vi "Fun gen and scope March 22 2017.vi"() -> ()   [LabVIEW 2014]
uses:
  <instrlib>/Tektronix TDS 200 1000 2000 Series/Public/Data/Read (Single Waveform).vi
  <vilib>/Utility/file.llb/Write To Spreadsheet File (string).vi
  <instrlib>/Stanford Research DS345/Stanford Research DS345.lvlib
  <instrlib>/Tektronix TDS 200 1000 2000 Series/Tektronix TDS 200 1000 2000 Series.lvlib
panel:
  out "File path":path
  in  "begin sweep":bool
  in  "End sweep now":bool
  in  "Manual control":T1={"Waveform"=1, "Amplitude (Vpp)"=4.0, "Frequency (Hz)"=1000.0, "Offset (V)"=3.25} {"Offset (V)" min=-3.25 max=3.25; "Frequency (Hz)" min=10.0 max=29000000.0 format="%#_8g"; "Amplitude (Vpp)" min=0.01 max=4.0; "Waveform" items=["Sine", "Square", "Triangle", "Ramp", "Noise"]}
  in  "Sweep control":T2={"Start amplitude (Vpp)"=0.05, "End amplitude (Vpp)"=4.0, "# of steps"=5.0, "# of scans at each ampl."=5.0} {"# of scans at each ampl." min=1.0 max=1000.0 step=1.0; "# of steps" min=1.0 max=1000.0 step=1.0; "End amplitude (Vpp)" min=0.01 max=4.0; "Start amplitude (Vpp)" min=0.01 max=8.0}
  out "Waveform Graph 2":waveform(dbl)(graph)
  out "Waveform Graph":waveform(dbl)(graph)
  in  "Stop Button":bool
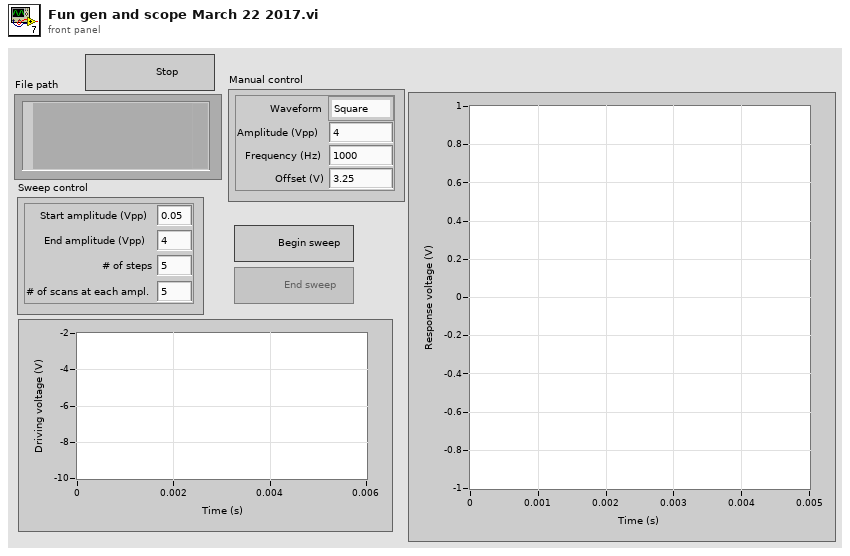
[diagram p1: front panel]
types:
  T1 = cluster{"Waveform":u16, "Amplitude (Vpp)":dbl, "Frequency (Hz)":dbl, "Offset (V)":dbl}
  T2 = cluster{"Start amplitude (Vpp)":dbl, "End amplitude (Vpp)":dbl, "# of steps":dbl, "# of scans at each ampl.":dbl}
  T3 = enum8{"Enabled", "Disabled", "Disabled and Grayed Out"}
  T4 = cluster{"Baud Rate":u32, "Parity":u16, "Data Bits":u16, "Stop Bits":u16, "Flow Control":u16}
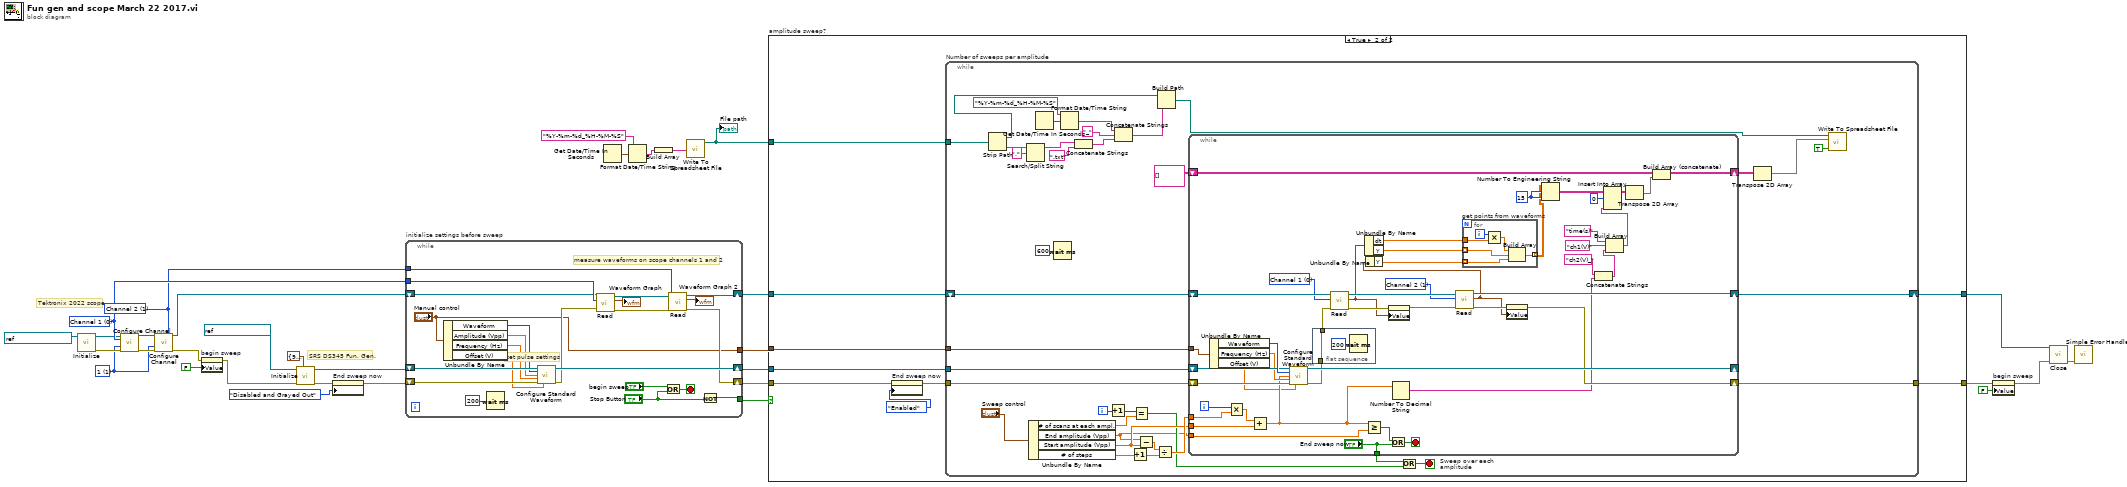
[diagram p0: block diagram]
diagram:
  w12 = 1 items=["1"=1, "10"=10, "20"=20, "50"=50, "100"=100, "500"=500, "1000"=1000] ("Probe Attenuation (10: 10X)")
  w15 = 0 items=["Channel 1", "Channel 2", "Channel 3", "Channel 4", "Math", "Reference A", "Reference B", "Reference C", "Reference D"] ("Channel (0: Channel 1)")
  w14 = 1 items=["Channel 1", "Channel 2", "Channel 3", "Channel 4", "Math", "Reference A", "Reference B", "Reference C", "Reference D"] ("Channel (0: Channel 1)")
  # "Tektronix 2022 scope"
  # "SRS DS345 Fun. Gen."
  n1 = call <instrlib>:"Initialize.vi"("VISA resource name"=refnum<visa-resource-name> "GPIB1::20::INSTR") -> ("error out"=w18:errorcluster, "VISA resource name out"=w13:refnum<visa-resource-name>)  [unwired: 9 in]
  n2 = call <instrlib>:"Configure Channel.vi"("VISA resource name"=w13, "Channel (0: Channel 1)"=w15, "Probe Attenuation (10: 10X)"=w12, "error in (no error)"=w18) -> ("VISA resource name out"=w19:refnum<visa-resource-name>, "error out"=w17:errorcluster)  [unwired: 10 in]
  n3 = call <instrlib>:"Configure Channel.vi"("VISA resource name"=w19, "Channel (0: Channel 1)"=w14, "Probe Attenuation (10: 10X)"=w12, "error in (no error)"=w17) -> ("VISA resource name out"=w16:refnum<visa-resource-name>, "error out"=w6:errorcluster)  [unwired: 10 in]
  n4 = property on="begin sweep" class="Bool (strict)"(error in=w6, "Value"=FALSE ("begin sweep")) -> (error out=w5:errorcluster)  [unwired: 1 in, 1 out]
  n5 = call <instrlib>:"Initialize.vi"("Serial Configuration"=T4 {"Baud Rate"=9600, "Parity"=0, "Data Bits"=8, "Stop Bits"=20, "Flow Control"=0}, "error in (no error)"=w5, "VISA resource name"=refnum<visa-resource-name> "GPIB2::19::INSTR") -> ("error out"=w25:errorcluster, "VISA resource name out"=w32:refnum<visa-resource-name>)  [unwired: 7 in]
  n6 = property on="End sweep now" class="Bool"(error in=w25, "DisabledEnum"=T3."Disabled and Grayed Out" ("Disabled")) -> (error out=w24:errorcluster)  [unwired: 1 in, 1 out]
  n7 = while "initialize settings before sweep" {
    shift-right: [w54] -> w30
    shift-left: w32 -> [w56]
    shift-right: [w36] -> w29
    shift-left: w24 -> [w55]
    tunnel: [w46] -> w23
    shift-right: [w40] -> w22
    shift-left: w16 -> [w41]
    tunnel: w15 -> [w45]
    tunnel: w14 -> [w44]
    tunnel: ["Manual control"] -> w9
    stop <- w48 stop-if-true
    # "measure waveforms on scope channels 1 and 2"
    # "set pulse settings"
    n8 = Unbundle By Name("Manual control") -> ("Waveform"=w52:u16, "Amplitude (Vpp)"=w51:dbl, "Frequency (Hz)"=w50:dbl, "Offset (V)"=w34:dbl)
    n9 = Wait (ms)(milliseconds to wait=u32 200) -> ()  [unwired: 1 out]
    n10 = call <instrlib>:"Configure Standard Waveform.vi"("VISA resource name"=w56, "Waveform Function (0: Sine)"=w52, "Amplitude (0.01 Vpp)"=w51, "Frequency (1000 Hz)"=w50, "error in (no error)"=w55, "DC Offset (0.00 V)"=w34) -> ("VISA resource name out"=w54:refnum<visa-resource-name>, "error out"=w37:errorcluster)  [unwired: 8 in]
    n11 = call-poly <instrlib>:"Read.vi"("error in (no error)"=w37, "Source (0: Channel 1)"=w45, "VISA resource name"=w41) -> ("error out"=w42:errorcluster, "Waveform Data"=→"Waveform Graph":waveform(dbl), "VISA resource name out"=w43:refnum<visa-resource-name>)  [unwired: 6 in]
    n12 = Or(x="begin sweep", y="Stop Button") -> (x .or. y?=w48:bool)
    n13 = call-poly <instrlib>:"Read.vi"("error in (no error)"=w42, "Source (0: Channel 1)"=w44, "VISA resource name"=w43) -> ("error out"=w36:errorcluster, "Waveform Data"=→"Waveform Graph 2":waveform(dbl), "VISA resource name out"=w40:refnum<visa-resource-name>)  [unwired: 6 in]
    n14 = Not(x="Stop Button") -> (.not. x?=w46:bool)
  }
  n15 = Get Date/Time In Seconds() -> (seconds since 1Jan1904=w4:timestamp)
  n16 = Format Date/Time String(time format string (%c)="%Y-%m-%d_%H-%M-%S", seconds (now)=w4) -> (date/time string=w3:string)  [unwired: 1 in]
  n17 = Build Array(w3) -> (w2:string[])
  n18 = call-poly <vilib>:"Write To Spreadsheet File.vi"("1D data"=w2) -> ("new file path (Not A Path if cancelled)"=w8:path)  [unwired: 7 in]
  "File path" <- w8
  n19 = case "amplitude sweep?" shown="True" w23 {
    tunnel: w30 -> [_ w67]
    tunnel: w29 -> [w58 w64]
    tunnel: [w58 w66] -> w27
    tunnel: w22 -> [w57 w62]
    tunnel: [w57 w61] -> w21
    tunnel: w9 -> [_ w60]
    tunnel: w8 -> [_ w59]
    frame False {
    }
    frame True {
      n20 = property on="End sweep now" class="Bool"(error in=w64, "DisabledEnum"=T3."Enabled" ("Disabled")) -> (error out=w63:errorcluster)  [unwired: 1 in, 1 out]
      n21 = while "Number of sweeps per amplitude" {
        tunnel: w67 -> [w104]
        tunnel: [w102] -> w66
        tunnel: w63 -> [w103]
        shift-right: [w95] -> w61
        shift-left: w62 -> [w96]
        tunnel: w60 -> [w91]
        tunnel: w59 -> [w69]
        i -> [w75]
        stop <- w92 stop-if-true
        n22 = Strip Path(path=w69) -> (stripped path=w70:path, name=w88:string)
        n23 = Search/Split String(string=w88, search string/char (-)=".") -> (substring before match=w83:string)  [unwired: 1 in, 2 out]
        n24 = Unbundle By Name("Sweep control") -> ("# of scans at each ampl."=w98:dbl, "End amplitude (Vpp)"=w89:dbl, "Start amplitude (Vpp)"=w99:dbl, "# of steps"=w78:dbl)
        n25 = Get Date/Time In Seconds() -> (seconds since 1Jan1904=w87:timestamp)
        n26 = Wait (ms)(milliseconds to wait=u32 600) -> ()  [unwired: 1 out]
        n27 = Format Date/Time String(time format string (%c)="%Y-%m-%d_%H-%M-%S", seconds (now)=w87) -> (date/time string=w73:string)  [unwired: 1 in]
        n28 = Concatenate Strings(w83, ".txt" ("string")) -> (w82:string)
        n29 = Increment(x=w75) -> (x+1=w97:i32)
        n30 = Concatenate Strings(w73, "_" ("string"), w82) -> (w81:string)
        n31 = Increment(x=w78) -> (x+1=w77:dbl)
        n32 = Equal?(x=w97, y=w98) -> (x = y?=w93:bool)
        n33 = Subtract(x=w89, y=w99) -> (x-y=w101:dbl)
        n34 = Divide(x=w101, y=w77) -> (x/y=w100:dbl)
        n35 = Build Path(base path=w70, name or relative path=w81) -> (appended path=w72:path)
        n36 = while "Sweep over each amplitude" {
          shift-right: [w147] -> _
          shift-left: w104 -> [w149]
          shift-right: [w130] -> w102
          shift-left: w103 -> [w148]
          tunnel: w91 -> [w131]
          tunnel: w100 -> [w145]
          tunnel: w99 -> [w144]
          shift-right: [w140] -> w95
          shift-left: w96 -> [w141]
          tunnel: ["End sweep now"] -> w94
          tunnel: w89 -> [w127]
          shift-right: [w119] -> w79
          shift-left: string[][] [] -> [w118]
          i -> [w108]
          stop <- w132 stop-if-true
          w124 = i16 15 ("precision (6)")
          w138 = 1 items=["Channel 1", "Channel 2", "Channel 3", "Channel 4", "Math", "Reference A", "Reference B", "Reference C", "Reference D"] ("Channel (0: Channel 1)")
          w139 = 0 items=["Channel 1", "Channel 2", "Channel 3", "Channel 4", "Math", "Reference A", "Reference B", "Reference C", "Reference D"] ("Channel (0: Channel 1)")
          n37 = Unbundle By Name(w131) -> ("Waveform"=w150:u16, "Frequency (Hz)"=w143:dbl, "Offset (V)"=w105:dbl)
          n38 = Multiply(x=w108, y=w145) -> (x*y=w146:dbl)
          n39 = Add(x=w146, y=w144) -> (x+y=w107:dbl)
          n40 = call <instrlib>:"Configure Standard Waveform.vi"("VISA resource name"=w149, "Waveform Function (0: Sine)"=w150, "Amplitude (0.01 Vpp)"=w107, "Frequency (1000 Hz)"=w143, "error in (no error)"=w148, "DC Offset (0.00 V)"=w105) -> ("VISA resource name out"=w147:refnum<visa-resource-name>, "error out"=w129:errorcluster)  [unwired: 8 in]
          n41 = flat-sequence {
            tunnel: w129 -> [w158]
            tunnel: [w158] -> w128
            frame #0 {
              n42 = Wait (ms)(milliseconds to wait=u32 200) -> ()  [unwired: 1 out]
            }
          }
          n43 = call-poly <instrlib>:"Read.vi"("error in (no error)"=w128, "Source (0: Channel 1)"=w139, "VISA resource name"=w141) -> ("error out"=w137:errorcluster, "Waveform Data"=w122:waveform(dbl), "VISA resource name out"=w142:refnum<visa-resource-name>)  [unwired: 6 in]
          n44 = Unbundle By Name(w122) -> ("dt"=w126:dbl, "Y"=w123:dbl[])
          n45 = Greater Or Equal?(x=w107, y=w127) -> (x >= y?=w134:bool)
          n46 = property on="Waveform Graph" class="WFGraph (strict)"(error in=w137, "Value"=w122) -> (error out=w136:errorcluster)  [unwired: 1 in, 1 out]
          n47 = Or(x=w134, y="End sweep now") -> (x .or. y?=w132:bool)
          n48 = Number To Decimal String(number=w107) -> (decimal integer string=w106:string)  [unwired: 1 in]
          n49 = call-poly <instrlib>:"Read.vi"("error in (no error)"=w136, "Source (0: Channel 1)"=w138, "VISA resource name"=w142) -> ("error out"=w135:errorcluster, "Waveform Data"=w121:waveform(dbl), "VISA resource name out"=w140:refnum<visa-resource-name>)  [unwired: 6 in]
          n50 = Unbundle By Name(w121) -> ("Y"=w125:dbl[])
          n51 = for "get points from waveforms" {
            tunnel: w126 -> [w155]
            tunnel: w123 -> [w153] mode=indexing
            tunnel: [w152] -> w120 mode=indexing
            tunnel: w125 -> [w151] mode=indexing
            i -> [w156]
            n52 = Multiply(x=w156, y=w155) -> (x*y=w154:dbl)
            n53 = Build Array(w154, w153, w151) -> (w152:dbl[])
          }
          n54 = property on="Waveform Graph 2" class="WFGraph (strict)"(error in=w135, "Value"=w121) -> (error out=w130:errorcluster)  [unwired: 1 in, 1 out]
          n55 = Number To Engineering String(2:w124, 3:w124, 4:w120) -> (0:w116:string[][])  [unwired: 1 in]
          n56 = Concatenate Strings("ch2(V)_", w106) -> (w109:string)
          n57 = Build Array("time(s)", "ch1(V)", w109) -> (w110:string[])
          n58 = Insert Into Array(array=w116, index (row)=0, new element=w110) -> (w115:string[][])  [unwired: 1 in]
          n59 = Transpose 2D Array(2D array=w115) -> (transposed array=w117:string[][])
          n60 = Build Array (concatenate)(w118, w117) -> (w119:string[][])
        }
        n61 = Or(x=w94, y=w93) -> (x .or. y?=w92:bool)
        n62 = Transpose 2D Array(2D array=w79) -> (transposed array=w76:string[][])
        n63 = call-poly <vilib>:"Write To Spreadsheet File.vi"("append to file? (new file:F)"=TRUE, "2D data"=w76, "file path (dialog if empty)"=w72) -> ()  [unwired: 5 in, 1 out]
      }
    }
  }
  n64 = property on="begin sweep" class="Bool (strict)"(error in=w27, "Value"=FALSE ("begin sweep")) -> (error out=w11:errorcluster)  [unwired: 1 in, 1 out]
  n65 = call <instrlib>:"Close.vi"("error in (no error)"=w11, "VISA resource name"=w21) -> ("error out"=w10:errorcluster)  [unwired: 9 in]
  n66 = call <vilib>:"Simple Error Handler.vi"("error in (no error)"=w10) -> ()  [unwired: 4 in, 5 out]
